vi "ReadIniFile.vi"(2 "Section":string="AzCamTool", 3 "key":string) -> (0 "found?":bool, 1 "value":string)   [LabVIEW 2014]
uses:
  globals/AzCamGlobals.vi
  <vilib>/Utility/config.llb/Read Key (String).vi
  <vilib>/Utility/config.llb/NI_LVConfig.lvlib
panel:
  out "appended path":path
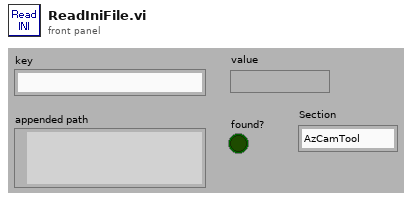
[diagram p1: front panel]
types:
  T1 = typedef "NI_LVConfig.lvlib/Config Data RefNum.ctl" = refnum<k1>
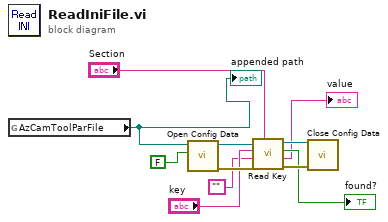
[diagram p0: block diagram]
diagram:
  n1 = global read "AzCamGlobals.vi" "AzCamToolParFile"() -> (w2:path)
  "appended path" <- w2
  n2 = call <vilib>:"Open Config Data.vi"("create file if necessary (T)"=FALSE ("create file if necessary? (T)"), "configuration file path"=w2) -> ("error out"=w9:errorcluster, "refnum"=w11:T1)  [unwired: 7 in, 1 out]
  n3 = call-poly <vilib>:"Read Key.vi"("section"="Section", "error in (no error)"=w9, "default value"="", "key"="key", "refnum"=w11) -> ("error out"=w7:errorcluster, "value"=→"value":string, "found?"=→"found?":bool, "refnum out"=w8:T1)  [unwired: 3 in]
  n4 = call <vilib>:"Close Config Data.vi"("error in (no error)"=w7, "refnum"=w8) -> ()  [unwired: 8 in, 2 out]
